vi "SP Get Value for Frequency.vi"(5 "Data":T1, 6 "Frequency (MHz)":dbl) -> (1 "Fractional Index":dbl, 2 "Value":dbl)   [LabVIEW 2011]
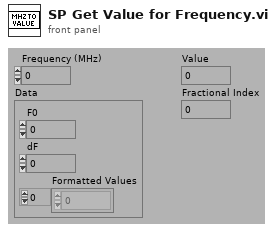
[diagram p1: front panel]
types:
  T1 = cluster{"F0":dbl, "dF":dbl, "Formatted Values":dbl[]}
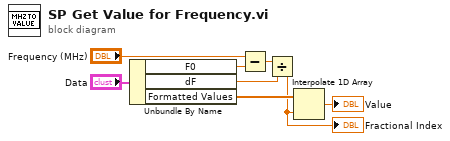
[diagram p0: block diagram]
diagram:
  n1 = Unbundle By Name("Data") -> ("F0"=w2:dbl, "dF"=w3:dbl, "Formatted Values"=w4:dbl[])
  n2 = Subtract(x="Frequency (MHz)", y=w2) -> (x-y=w6:dbl)
  n3 = Divide(x=w6, y=w3) -> (x/y=w1:dbl)
  "Fractional Index" <- w1
  n4 = Interpolate 1D Array(1:w1, 2:w4) -> (0:→"Value":dbl)
